vi "RSZVB Set Simultaneous Measurement Of Ports Groups.vi"(8 "error in (no error)":errorcluster {"code" format="%.0x"}, 9 "State (On)":bool=TRUE, 10 "Channel (1)":i32=1, 11 "VISA resource name":refnum<visa-resource-name>) -> (0 "error out":errorcluster {"code" format="%.0x"}, 3 "VISA resource name out":refnum<visa-resource-name>)   [LabVIEW 2011]
doc: "This VI activates/deactivates simultaneous measurement of port groups. Please note that setting this flag does not change the port group setup. \n\n\nNote(s):\n\n(1) Simultaneous Measurement of Port Groups is not available in any one of the following situations:\n\n- Less than two port groups are defined \n- Frequency Converter mode is active\n- True Differential Mode or Defined Coherence Mode is active\n- In a frequency converting measurement where Measure Source Port Waves at: Source Frequency is chosen in the Port Configuration.\n\nRemote-control command(s):\nSOURce<Ch>:GROup:SIMultaneous:STATe"
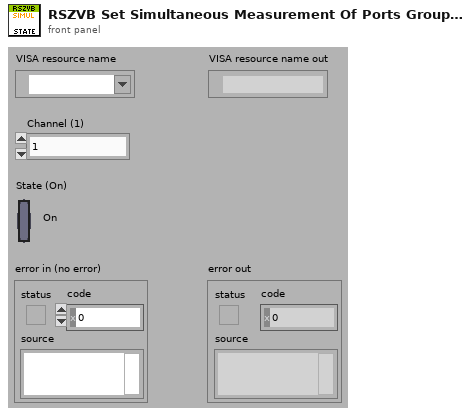
[diagram p1: front panel]
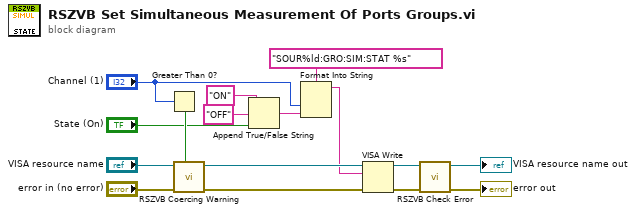
[diagram p0: block diagram]
diagram:
  n1 = Greater Than 0?(x="Channel (1)") -> (x > 0?=w10:bool)
  n2 = call "RSZVB Coercing Warning.vi"("In Range?"=w10, "error in (no error)"="error in (no error)", "VISA session"="VISA resource name") -> ("error out"=w14:errorcluster, "dup VISA session"=w15:refnum<visa-resource-name>)  [unwired: 7 in]
  n3 = Append True/False String(1:"State (On)", 2:"OFF", 3:"ON") -> (0:w7:string)  [unwired: 1 in]
  n4 = Format Into String(format string="SOUR%ld:GRO:SIM:STAT %s", "Channel (1)", w7) -> (resulting string=w11:string)  [unwired: 2 in, 1 out]
  n5 = VISA Write(VISA resource name=w15, write buffer=w11, error in (no error)=w14) -> (VISA resource name out=w12:refnum<visa-resource-name>, error out=w13:errorcluster)  [unwired: 1 out]
  n6 = call "RSZVB Check Error.vi"("error in (no error)"=w13, "VISA session"=w12) -> ("error out"=→"error out":errorcluster, "dup VISA session"=→"VISA resource name out":refnum<visa-resource-name>)  [unwired: 8 in]
